vi "test_Error Code and Message Status Channels by Generating Protection Error (-265).vi"(8 "error in (no error)":errorcluster, 11 "TestCase in":refnum<class "Instrument Addon Error System Tests.lvclass">) -> (0 "error out":errorcluster, 3 "TestCase out":refnum<class "Instrument Addon Error System Tests.lvclass">)   [LabVIEW 2019, in "Instrument Addon Error System Tests.lvclass"]
uses:
  Instrument Addon Error System Tests.lvclass
  C:/Program Files (x86)/National Instruments/LabVIEW 2019/vi.lib/NI/VeriStand Custom Device Testing Tools/VeriStandTestCase/VeriStandTestCase.lvclass
  <vilib>/NI VeriStand/Execution/Workspace/NI VeriStand - Get Multiple Channel Values.vi
  <vilib>/NI VeriStand/Execution/Workspace/NI VeriStand - Set Multiple Channel Values.vi
  <vilib>/addons/_JKI Toolkits/VI Tester/TestCase.llb/TestCase.lvclass
  <vilib>/NI VeriStand/Execution/Workspace/NI_VS Workspace ExecutionAPI.lvlib
  C:/Program Files (x86)/National Instruments/LabVIEW 2019/vi.lib/addons/_JKI Toolkits/VI Tester/TestCase.llb/TestCase.lvclass
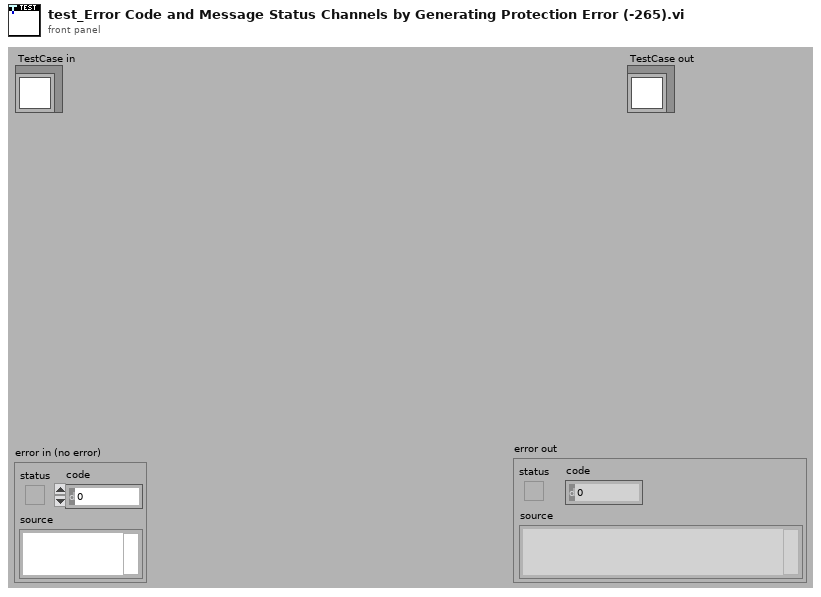
[diagram p1: front panel]
types:
  T1 = typedef "NI_VS Workspace ExecutionAPI.lvlib/WorkspaceAPI.ctl" = refnum<k24>
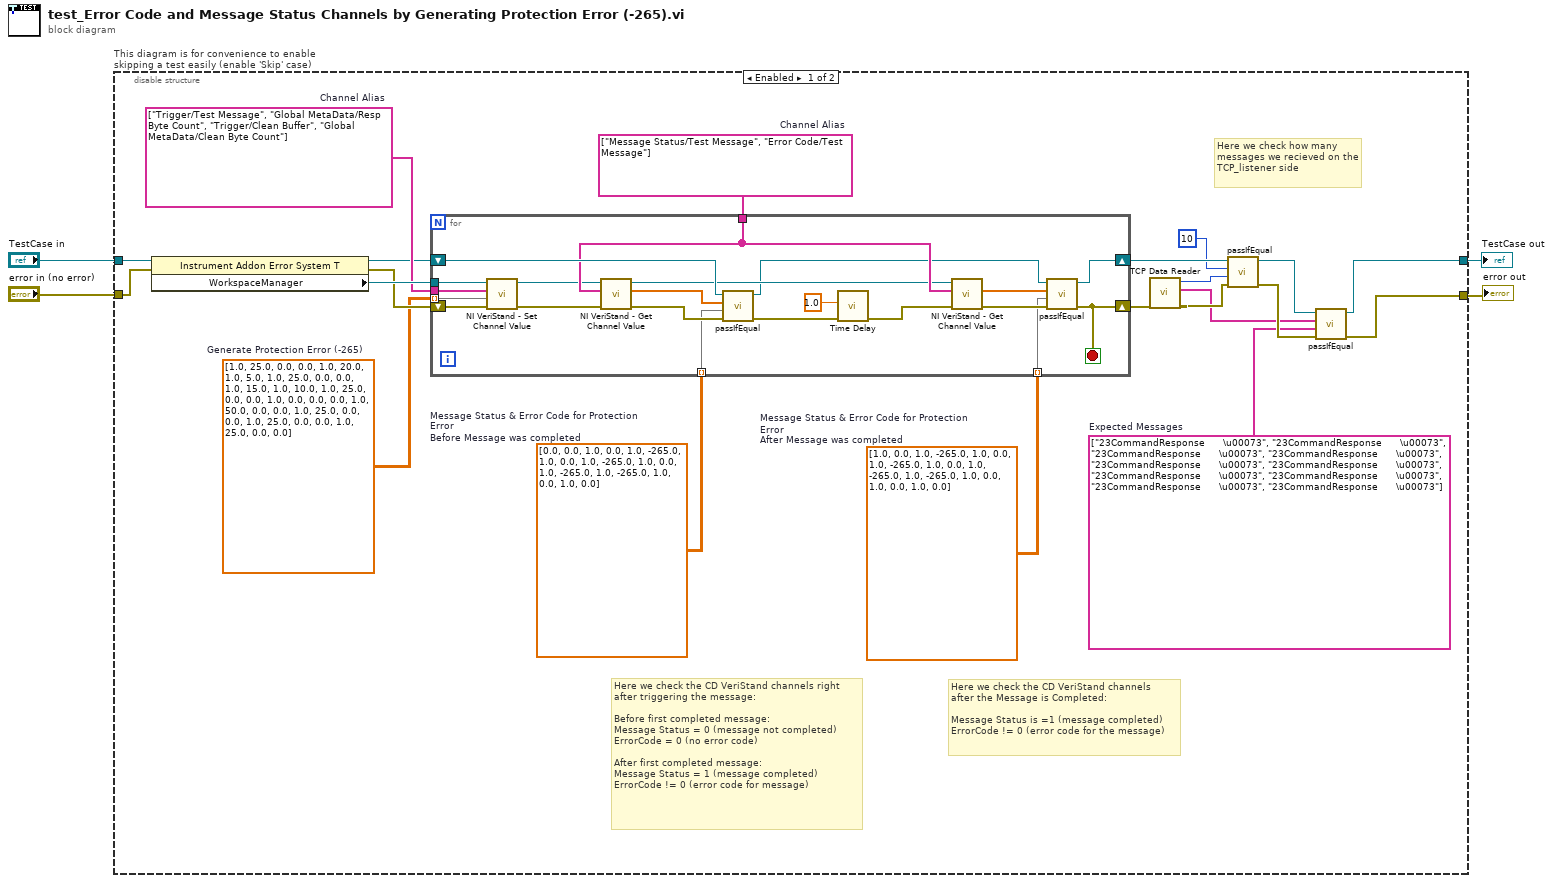
[diagram p0: block diagram]
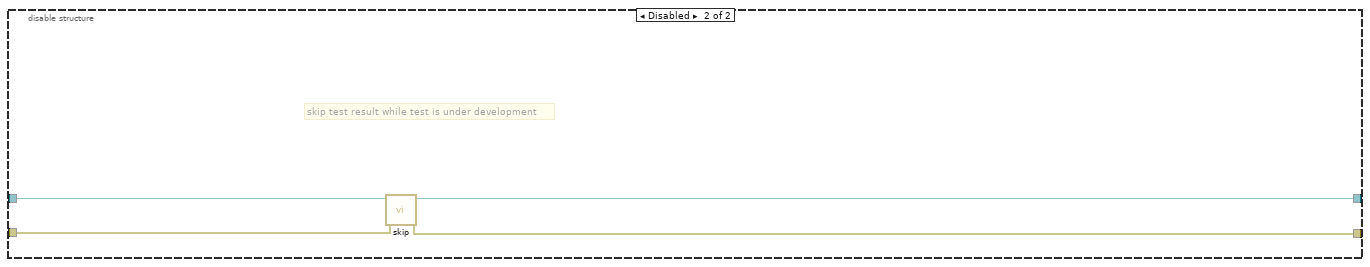
[diagram p2: hidden frame]
diagram:
  n1 = disable-structure "This diagram is for convenience to enable skipping a test easily (enable 'Skip' case)" shown="Enabled" {
    disable-tunnel: "TestCase in" -> [w25 w50]
    disable-tunnel: [w18 w48] -> w1
    disable-tunnel: [w16 w49] -> w3
    disable-tunnel: "error in (no error)" -> [w24 w47]
    frame Enabled {
      w5 = dbl[][] [[1.0, 0.0], [1.0, -265.0], [1.0, 0.0], [1.0, -265.0], [1.0, 0.0], [1.0, -265.0], [1.0, -265.0], [1.0, 0.0], [1.0, 0.0], [1.0, 0.0]]  # Message Status & Error Code for Protection Error After Message was completed
      w6 = dbl[][] [[0.0, 0.0], [1.0, 0.0], [1.0, -265.0], [1.0, 0.0], [1.0, -265.0], [1.0, 0.0], [1.0, -265.0], [1.0, -265.0], [1.0, 0.0], [1.0, 0.0]]  # Message Status & Error Code for Protection Error Before Message was completed
      w7 = dbl[][] [[1.0, 25.0, 0.0, 0.0], [1.0, 20.0, 1.0, 5.0], [1.0, 25.0, 0.0, 0.0], [1.0, 15.0, 1.0, 10.0], [1.0, 25.0, 0.0, 0.0], [1.0, 0.0, 0.0, 0.0], [1.0, 50.0, 0.0, 0.0], [1.0, 25.0, 0.0, 0.0], [1.0, 25.0, 0.0, 0.0], [1.0, 25.0, 0.0, 0.0]]  # Generate Protection Error (-265)
      w14 = string[] ["23CommandResponse      \u00073", "23CommandResponse      \u00073", "23CommandResponse      \u00073", "23CommandResponse      \u00073", "23CommandResponse      \u00073", "23CommandResponse      \u00073", "23CommandResponse      \u00073", "23CommandResponse      \u00073", "23CommandResponse      \u00073", "23CommandResponse      \u00073"]  # Expected Messages
      w8 = string[] ["Message Status/Test Message", "Error Code/Test Message"]  # Channel Alias
      w21 = string[] ["Trigger/Test Message", "Global MetaData/Resp Byte Count", "Trigger/Clean Buffer", "Global MetaData/Clean Byte Count"]  # Channel Alias
      # "Here we check the CD VeriStand channels right\nafter triggering the message:\n\nBefore first completed message:\nMessage Status = 0 (message not completed)\nErrorCode = 0 (no error code)\n\nAfter first completed message:\nMessage Status = 1 (message completed)\nErrorCode != 0 (error code for message)"
      # "Here we check how many messages we recieved on the TCP_listener side"
      # "Here we check the CD VeriStand channels\nafter the Message is Completed:\n\nMessage Status is =1 (message completed)\nErrorCode != 0 (error code for the message)"
      n2 = property class="Instrument Addon Error System T"(reference=w25, error in=w24) -> (reference out=w20:refnum<class "Instrument Addon Error System Tests.lvclass">, error out=w22:errorcluster, "WorkspaceManager"=w23:T1)
      n3 = for {
        tunnel: w23 -> [w46]
        tunnel: w21 -> [w44]
        tunnel: w8 -> [w41]
        tunnel: w7 -> [w40] mode=indexing
        shift-right: [w26] -> w12
        shift-left: w22 -> [w45]
        shift-right: [w42] -> w15
        shift-left: w20 -> [w43]
        tunnel: w6 -> [w29] mode=indexing
        tunnel: w5 -> [w28] mode=indexing
        stop <- w26 stop-if-true
        n4 = call-poly <vilib>:"NI VeriStand - Set Channel Value.vi"("error in (no error)"=w45, "Values"=w40, "Channels"=w44, "WorkspaceManager in"=w46) -> ("error out"=w34:errorcluster, "WorkspaceManager out"=w36:T1)  [unwired: 6 in]
        n5 = call-poly <vilib>:"NI VeriStand - Get Channel Value.vi"("error in (no error)"=w34, "Channels"=w41, "WorkspaceManager in"=w36) -> ("error out"=w32:errorcluster, "Values"=w31:dbl[], "WorkspaceManager out"=w35:T1)  [unwired: 6 in]
        n6 = call-dynamic "passIfEqual.vi"("error in (no error)"=w32, "y"=w29, "x"=w31, "TestCase in"=w43) -> ("error out"=w27:errorcluster, "TestCase out"=w33:refnum<class "Instrument Addon Error System Tests.lvclass">)  [unwired: 6 in]
        n7 = call "Time Delay"("error in (no error)"=w27, "Delay Time (s)"=1.0) -> ("error out"=w38:errorcluster)  [unwired: 9 in]
        n8 = call-poly <vilib>:"NI VeriStand - Get Channel Value.vi"("error in (no error)"=w38, "Channels"=w41, "WorkspaceManager in"=w35) -> ("error out"=w37:errorcluster, "Values"=w30:dbl[])  [unwired: 6 in, 1 out]
        n9 = call-dynamic "passIfEqual.vi"("error in (no error)"=w37, "y"=w28, "x"=w30, "TestCase in"=w33) -> ("error out"=w26:errorcluster, "TestCase out"=w42:refnum<class "Instrument Addon Error System Tests.lvclass">)  [unwired: 6 in]
      }
      n10 = call "TCP Data Reader.vi"("error in (no error)"=w12) -> ("error out"=w10:errorcluster, "Recieved Messages"=w9:string[], "No of messages"=w11:i32)  [unwired: 8 in]
      n11 = call-dynamic "passIfEqual.vi"("error in (no error)"=w10, "y"=w11, "x"=10 ("Expected no of messages"), "TestCase in"=w15) -> ("error out"=w17:errorcluster, "TestCase out"=w19:refnum<class "Instrument Addon Error System Tests.lvclass">)  [unwired: 6 in]
      n12 = call-dynamic "passIfEqual.vi"("error in (no error)"=w17, "y"=w14, "x"=w9, "TestCase in"=w19) -> ("error out"=w16:errorcluster, "TestCase out"=w18:refnum<class "Instrument Addon Error System Tests.lvclass">)  [unwired: 6 in]
    }
    frame Disabled {
      # "skip test result while test is under development"
      n13 = call <vilib>:"skip.vi"("error in (no error)"=w47, "TestCase in"=w50) -> ("error out"=w49:errorcluster, "TestCase out"=w48:refnum<class "Instrument Addon Error System Tests.lvclass">)  [unwired: 8 in]
    }
  }
  "error out" <- w3
  "TestCase out" <- w1
